vi "From Serial Form.vi"(6 "Serial Version":T1, 10 "Deserializer in":refnum<class "Deserializer.lvclass">, 11 "CRDS Cell in":refnum<class "CRDS Cell.lvclass">) -> (0 "error out":errorcluster, 2 "Deserializer out":refnum<class "Deserializer.lvclass">, 3 "CRDS Cell out":refnum<class "CRDS Cell.lvclass">)   [LabVIEW 2012, in "CRDS Cell.lvclass"]
uses:
  CRDS Cell.lvclass
  <userlib>/Serialization/Deserializer/Deserializer.lvclass
  <userlib>/Serialization/Serialization Common/Serial Version.ctl
  <userlib>/Serialization/Serializable/Serializable.lvclass
  Get Tau Method.ctl
  CRDS Cell.lvclass/CRDS Cell.ctl
  <userlib>/Serialization/Serializable/Remove Single.vi
  <userlib>/Serialization/Serializable/Remove Boolean.vi
  <userlib>/Serialization/Serializable/Remove Double.vi
  <userlib>/Serialization/Serializable/Remove Int08.vi
  <userlib>/Serialization/Serializable/Remove UInt08.vi
  <userlib>/Serialization/Serialization Common/Serialization Common.lvlib
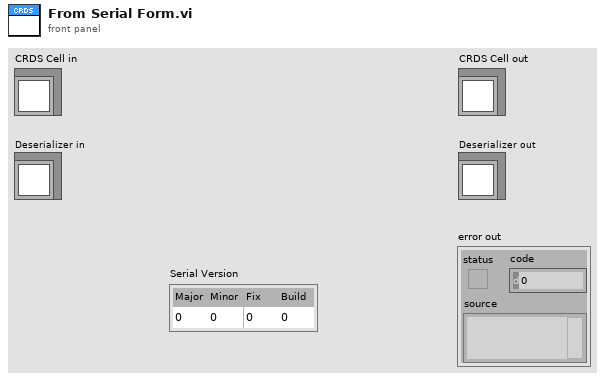
[diagram p1: front panel]
types:
  T1 = typedef "Serialization Common.lvlib/Serial Version.ctl" = cluster{"Major":u16, "Minor":u16, "Fix":u16, "Build":u16}
  T2 = typedef "Get Tau Method.ctl" = enum8{"DFT-1", "DFT-5", "LRS"}
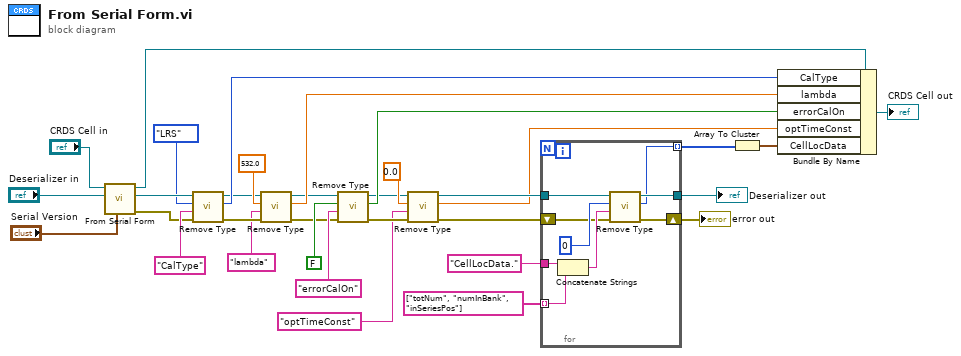
[diagram p0: block diagram]
diagram:
  n1 = call-parent "From Serial Form.vi"("Serial Version"="Serial Version", "Deserializer in"="Deserializer in", "Serializable in"="CRDS Cell in") -> ("error out"=w22:errorcluster, "Deserializer out"=w29:refnum<class "Deserializer.lvclass">, "Serializable out"=w30:refnum<class "CRDS Cell.lvclass">)  [unwired: 6 in]
  n2 = call-poly <userlib>:"Remove Type.vi"("error in (no error)"=w22, "Name"="CalType", "Default Value"=Get_Tau_Method."LRS" ("CalType"), "Deserializer in"=w29) -> ("error out"=w23:errorcluster, "Numeric"=w26:i8, "Deserializer out"=w24:refnum<class "Deserializer.lvclass">)  [unwired: 4 in, 1 out]
  n3 = call-poly <userlib>:"Remove Type.vi"("error in (no error)"=w23, "Name"="lambda", "Default Value"=532.0 ("lambda"), "Deserializer in"=w24) -> ("error out"=w1:errorcluster, "Numeric"=w21:dbl, "Deserializer out"=w18:refnum<class "Deserializer.lvclass">)  [unwired: 4 in, 1 out]
  n4 = call-poly <userlib>:"Remove Type.vi"("error in (no error)"=w1, "Name"="errorCalOn", "Default Value"=FALSE ("errorCalOn"), "Deserializer in"=w18) -> ("error out"=w12:errorcluster, "Boolean"=w15:bool, "Deserializer out"=w13:refnum<class "Deserializer.lvclass">)  [unwired: 4 in, 1 out]
  n5 = call-poly <userlib>:"Remove Type.vi"("error in (no error)"=w12, "Name"="optTimeConst", "Default Value"=sgl 0.0 ("optTimeConst"), "Deserializer in"=w13) -> ("error out"=w2:errorcluster, "Numeric"=w6:sgl, "Deserializer out"=w8:refnum<class "Deserializer.lvclass">)  [unwired: 4 in, 1 out]
  n6 = for {
    tunnel: w8 -> [w40]
    tunnel: string[] ["totNum", "numInBank", "inSeriesPos"] -> [w42] mode=indexing
    tunnel: "CellLocData." ("Name") -> [w41]
    tunnel: [w39] -> w4
    shift-right: [w36] -> w3
    shift-left: w2 -> [w35]
    tunnel: [w34] -> w7 mode=indexing
    n7 = Concatenate Strings(w41, w42) -> (w37:string)
    n8 = call-poly <userlib>:"Remove Type.vi"("error in (no error)"=w35, "Name"=w37, "Default Value"=u8 0, "Deserializer in"=w40) -> ("error out"=w36:errorcluster, "Numeric"=w34:u8, "Deserializer out"=w39:refnum<class "Deserializer.lvclass">)  [unwired: 4 in, 1 out]
  }
  "error out" <- w3
  "Deserializer out" <- w4
  n9 = Array To Cluster(array=w7) -> (cluster=w5:cluster{"[0]":u8, "[1]":u8, "[2]":u8})
  n10 = Bundle By Name(cluster=w30, "CalType"=w26, "lambda"=w21, "errorCalOn"=w15, "optTimeConst"=w6, "CellLocData"=w5) -> (→"CRDS Cell out":refnum<class "CRDS Cell.lvclass">)
